vi "habLogic.vi"(5 "Climb button":bool, 7 "Retract Button":bool, 11 "Safety Button":bool) -> (1 "Retract and Safety Pressed?":bool, 2 "Climb and Safety Pressed?":bool, 3 "Hab state":string)   [LabVIEW 2018]
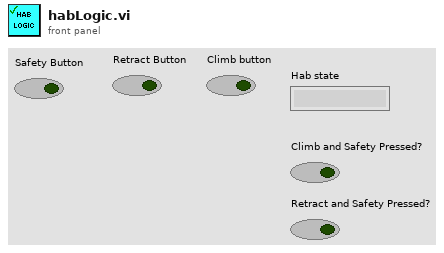
[diagram p1: front panel]
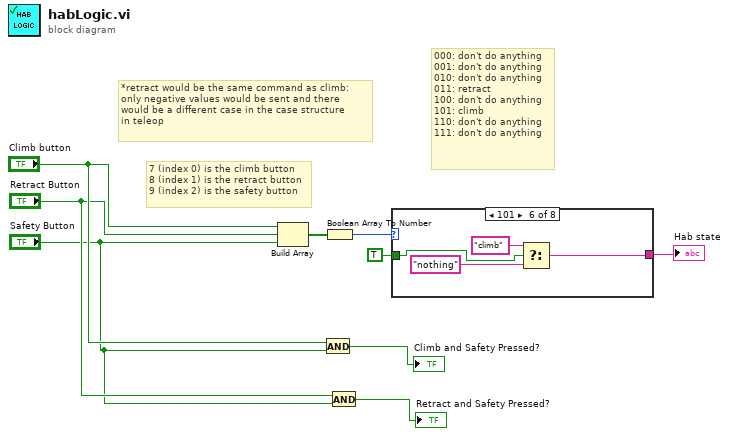
[diagram p0: block diagram]
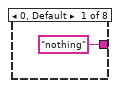
[diagram p2: hidden frame]
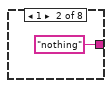
[diagram p3: hidden frame]
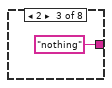
[diagram p4: hidden frame]
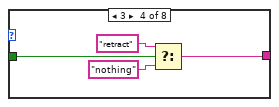
[diagram p5: hidden frame]
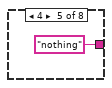
[diagram p6: hidden frame]
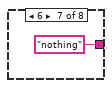
[diagram p7: hidden frame]
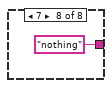
[diagram p8: hidden frame]
diagram:
  # "*retract would be the same command as climb:\nonly negative values would be sent and there\nwould be a different case in the case structure\nin teleop"
  # "7 (index 0) is the climb button\n8 (index 1) is the retract button\n9 (index 2) is the safety button"
  # "000: don't do anything\n001: don't do anything\n010: don't do anything\n011: retract\n100: don't do anything\n101: climb\n110: don't do anything\n111: don't do anything"
  n1 = Build Array("Climb button", "Retract Button", "Safety Button") -> (w9:bool[])
  n2 = And(x="Climb button", y="Safety Button") -> (x .and. y?=→"Climb and Safety Pressed?":bool)
  n3 = Boolean Array To Number(Boolean array=w9) -> (number=w8:u32)
  n4 = And(x="Retract Button", y="Safety Button") -> (x .and. y?=→"Retract and Safety Pressed?":bool)
  n5 = case shown="101" w8 {
    tunnel: TRUE -> [_ _ _ w16 _ w18 _ _]
    tunnel: ["nothing" ("f") "nothing" ("f") "nothing" ("f") w13 "nothing" ("f") w19 "nothing" ("f") "nothing" ("f")] -> w7
    frame 0, Default {
    }
    frame 1 {
    }
    frame 2 {
    }
    frame 3 {
      n6 = Select(t="retract", s=w16, f="nothing") -> (s? t:f=w13:string)
    }
    frame 4 {
    }
    frame 5 {
      n7 = Select(t="climb", s=w18, f="nothing") -> (s? t:f=w19:string)
    }
    frame 6 {
    }
    frame 7 {
    }
  }
  "Hab state" <- w7
